vi "Internet Connection Monitor.vi"() -> ()   [LabVIEW 2023]
doc: "This VI pings google.com every 1000mS and waits 500mS for a response."
uses:
  <vilib>/Platform/TimedLoop/XDataNode/timing_clust.ctl
  <vilib>/Platform/TimedLoop/XDataNode/nitl_modes.ctl
  <vilib>/Platform/TimedLoop/XDataNode/wakeup.ctl
  Type Definitions/Internet Connection Monitor.ctl
  Type Definitions/Payload Class.ctl
  Type Definitions/Enumerated Constants/Software Monitor.ctl
  <vilib>/platform/TimedLoop/XDataNode/XDataNode.xnode
  <vilib>/Platform/TimedLoop/XDataNode/XDNodeRunTimeDep.lvlib
panel:
  out "standard output 4":string
  out "after substring 2":string
  out "offset past match 2":i32
  out "Connected to world wide web? 2":bool
  out "error out 2":errorcluster
  out "standard error 2":string
  out "Numeric 2":i32
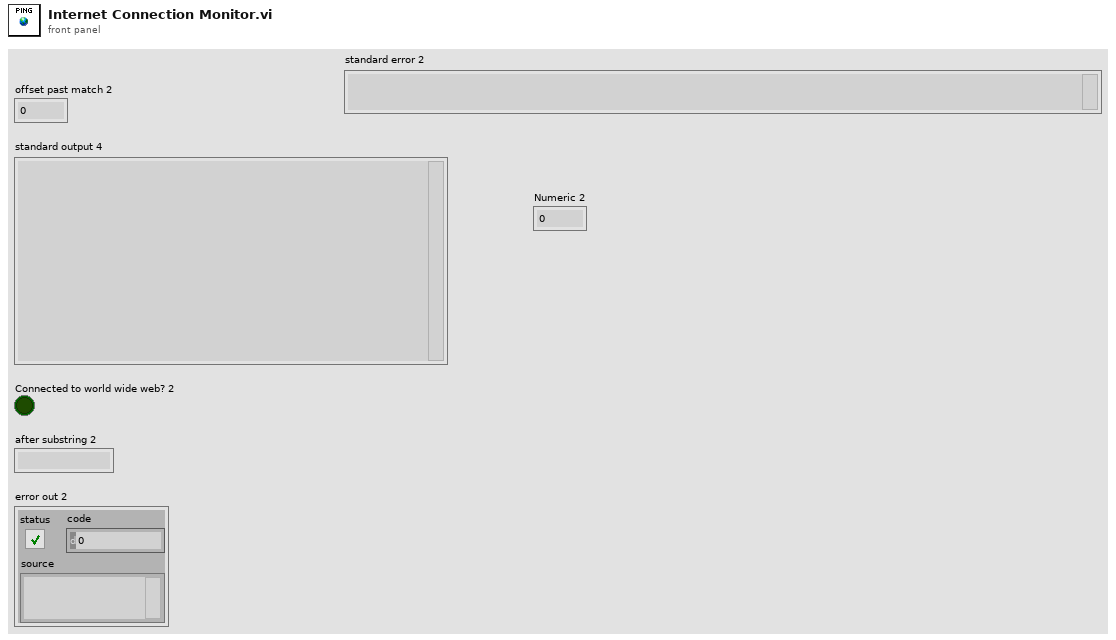
[diagram p1: front panel]
types:
  T1 = typedef "XDNodeRunTimeDep.lvlib/timing_clust.ctl" = cluster{"Expected End [f-1]":u64, "Actual End [f-1]":u64, "Finished Late? [f-1]":bool, "Expected End [i-1]":u64, "Actual End [i-1]":u64, "Finished Late? [i-1]":bool, "Expected Start [i]":u64, "Actual Start [i]":u64, "Expected Start [f]":u64, "Actual Start [f]":u64, "Source Name":string, "Structure Name":string, "Period":i64, "Deadline":i64, "Offset":i64, "Start":i64, "Priority":i32, "Timeout":i32, "Mode":T2, "Wakeup Reason":T3, "Error":errorcluster, "Source Type":string, "Secondary Source Type":string, "Global End Time":u64, "Global Start Time":u64, "Frame Duration":u64, "Iteration Duration":u64, "Assigned CPU":i32, "I/O Scan Engine Mode":u32}
  T2 = typedef "XDNodeRunTimeDep.lvlib/nitl_modes.ctl" = enum32{"No Change", "Process missed periods, maintain original phase", "Discard missed periods, maintain original phase", "Process missed periods, ignore original phase", "Discard missed periods, ignore original phase"}
  T3 = typedef "XDNodeRunTimeDep.lvlib/wakeup.ctl" = enum32{"Normal", "Aborted", "Asynchronous wakeup", "Timing source error", "Timed loop error", "Timeout"}
  T4 = typedef "Software Monitor.ctl" = enum16{"Internet Connection Monitor", "CPU Monitor", "Archive Monitor", "Memory Monitor", "Queue Monitor", "RTOS Update", "RTOS Monitor"}
  T5 = typedef "Payload Class.ctl" = enum16{"System State", "Parameters", "Metadata", "Software Monitor", "Data", "Commands"}
  T6 = typedef "Internet Connection Monitor.ctl" = cluster{"Connected?":bool, "Ping Latency (uS)":i32, "Ping Address":string}
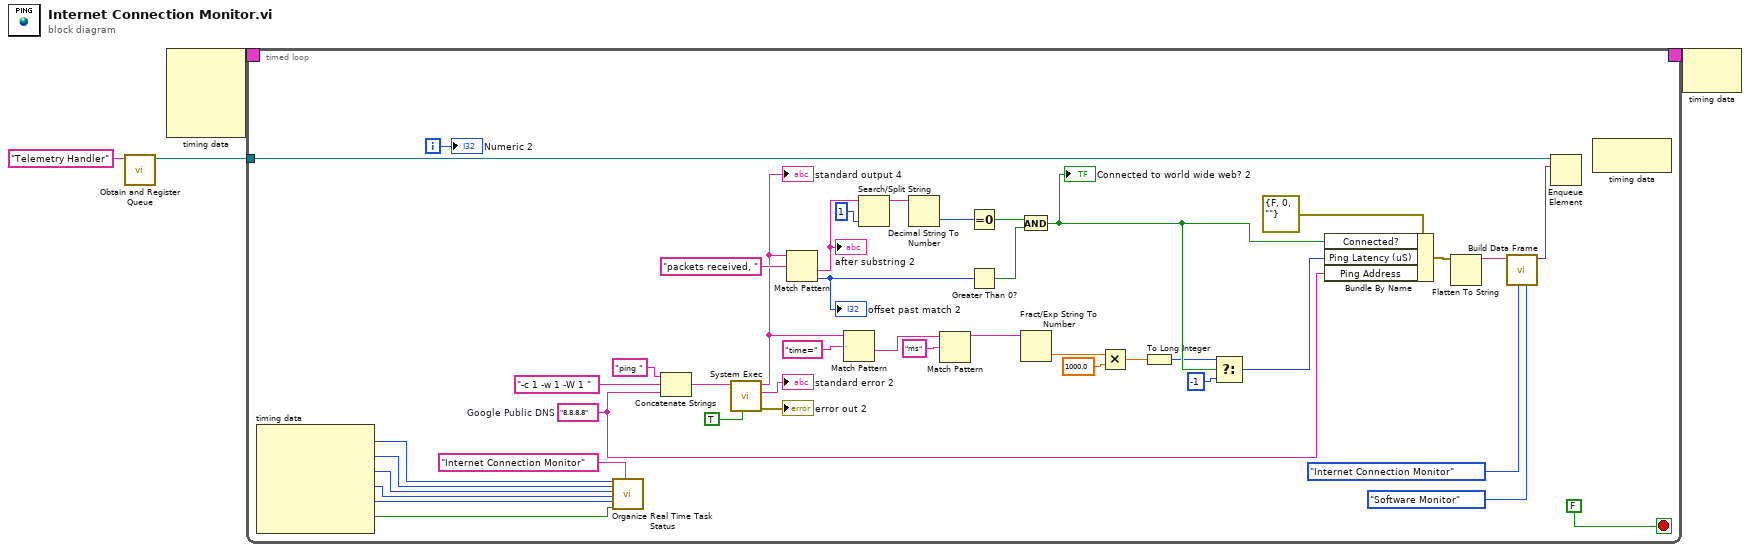
[diagram p0: block diagram]
diagram:
  n1 = call "Obtain and Register Queue.vi"("Queue Name (unnamed)"="Telemetry Handler" ("name (unnamed)")) -> ("Queue Reference"=w1:refnum<queue>)  [unwired: 9 in, 1 out]
  n2 = node-c288() -> (w4:T1)  [unwired: 4 in]
  n3 = timed-loop {
    tunnel: w1 -> [w31]
    timing: w4 -> [_]
    timing-out: [_] -> w3
    i -> [w6]
    stop <- FALSE stop-if-true
    w8 = "8.8.8.8"  # Google Public DNS
    n4 = node-c288() -> (w15:i32, w14:i32, w13:i64, w12:i64, w11:i64, w10:bool)  [unwired: 1 in]
    n5 = call "Organize Real Time Task Status.vi"("Priority"=w15, "Processor"=w14, "Offset"=w13, "Iteration Duration"=w12, "Period"=w11, "Finished Late? [i-1]"=w10, "Task Name"="Internet Connection Monitor") -> ()  [unwired: 12 in, 1 out]
    n6 = Concatenate Strings("ping " ("string"), "-c 1 -w 1 -W 1 " ("string"), w8) -> (w5:string)
    n7 = call <vilib>:"System Exec.vi"("run minimized? (F)"=TRUE, "command line"=w5) -> ("error out"=→"error out 2":errorcluster, "standard error"=→"standard error 2":string, "standard output"=w29:string)  [unwired: 6 in, 1 out]
    "standard output 4" <- w29
    n8 = Match Pattern(string=w29, regular expression="packets received, " ("search string/char (-)")) -> (after substring=w44:string, offset past match=w39:i32)  [unwired: 1 in, 2 out]
    "after substring 2" <- w44
    "offset past match 2" <- w39
    n9 = Match Pattern(string=w29, regular expression="time=" ("search string/char (-)")) -> (after substring=w27:string)  [unwired: 1 in, 3 out]
    n10 = Search/Split String(string=w44, offset (0)=1) -> (substring before match=w42:string)  [unwired: 1 in, 2 out]
    n11 = Decimal String To Number(string=w42) -> (number=w41:i32)  [unwired: 2 in, 1 out]
    n12 = Match Pattern(string=w27, regular expression="ms" ("search string/char (-)")) -> (before substring=w26:string)  [unwired: 1 in, 3 out]
    n13 = Equal To 0?(x=w41) -> (x = 0?=w37:bool)
    n14 = Greater Than 0?(x=w39) -> (x > 0?=w38:bool)
    n15 = And(x=w37, y=w38) -> (x .and. y?=w20:bool)
    "Connected to world wide web? 2" <- w20
    n16 = Fract/Exp String To Number(string=w26) -> (number=w25:dbl)  [unwired: 3 in, 1 out]
    n17 = Multiply(x=w25, y=1000.0) -> (x*y=w23:dbl)
    n18 = To Long Integer(number=w23) -> (32bit integer=w19:i32)
    n19 = Select(t=w19, s=w20, f=-1) -> (s? t:f=w17:i32)
    n20 = Bundle By Name(cluster=T6 {"Connected?"=FALSE, "Ping Latency (uS)"=0, "Ping Address"=""}, "Connected?"=w20, "Ping Latency (uS)"=w17, "Ping Address"=w8) -> (w33:T6)
    n21 = Flatten To String(anything=w33) -> (data string=w36:string)  [unwired: 3 in, 2 out]
    n22 = call "Build Data Frame.vi"("Payload Class (Data)"=Payload_Class."Software Monitor", "Payload ID (0)"=Software_Monitor."Internet Connection Monitor", "Payload (Empty String)"=w36) -> ("Frame"=w35:variant)  [unwired: 7 in, 1 out]
    n23 = Enqueue Element(queue=w31, element=w35) -> ()  [unwired: 2 in, 3 out]
    n24 = node-c288() -> ()  [unwired: 1 in, 1 out]
    "Numeric 2" <- w6
  }
  n25 = node-c288(w3) -> ()  [unwired: 1 out]
